vi "Build UDP Payload.vi"(8 "error in (no error)":errorcluster, 11 "DiscoveryService in":refnum<class "NodeDiscovery.lvclass">) -> (0 "error out":errorcluster, 2 "UDP Payload":string, 3 "DiscoveryService out":refnum<class "NodeDiscovery.lvclass">)   [LabVIEW 2020, in "Vecto.lvlib" / "NodeDiscovery.lvclass"]
uses:
  NodeDiscovery.lvclass
  NodeDiscovery.lvclass/NodeDiscovery.ctl
  Vecto.lvlib
  proto/Discovery/Class/Msg.lvclass
  C:/dev/lv20CE/lv-vecto/Vecto/proto/Discovery/Class/Msg.lvclass
  C:/Program Files (x86)/National Instruments/LabVIEW 2020/vi.lib/IlluminatedG/IG Protoc/LV-Proto/Message/Message.lvclass
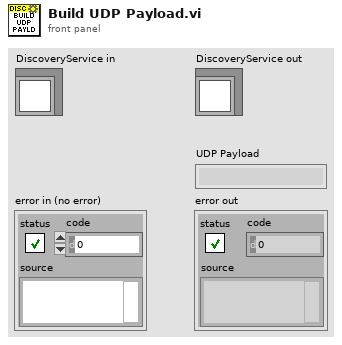
[diagram p1: front panel]
types:
  T1 = typedef "Discovery.lvlib/Data.ctl" = cluster{"node_id":u32, "name":string, "ip":u32, "status":string, "services":T2[], "system":string, "cluster":string}
  T2 = typedef "Service.lvlib/Data.ctl" = cluster{"type":T3, "port":i32}
  T3 = typedef "ServiceType.lvlib/Enumeration.ctl" = enum16{"SERVICETYPE_UNKNOWN", "SERVICETYPE_TCPSERVER", "SERVICETYPE_HTTPSERVER"}
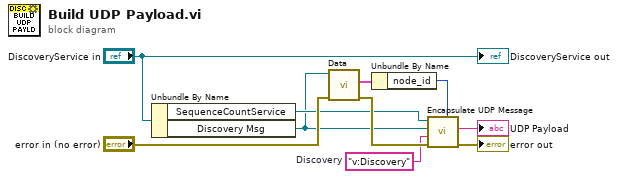
[diagram p0: block diagram]
diagram:
  w1 = "v:Discovery"  # Discovery
  n1 = Unbundle By Name("DiscoveryService in") -> ("SequenceCountService"=w8:refnum<class "SequenceCountService.lvclass">, "Discovery Msg"=w7:refnum<class "Msg.lvclass">)
  n2 = call "Data.vi"("error in (no error)"="error in (no error)", "PB Msg Template in"=w7) -> ("error out"=w10:errorcluster, "Data"=w6:T1)  [unwired: 7 in, 1 out]
  n3 = Unbundle By Name(w6) -> ("node_id"=w5:u32)
  n4 = call "Encapsulate UDP Message.vi"("source_id"=w5, "error in (no error)"=w10, "type"=w1, "Encapsulated Msg"=w7, "SequenceCountService"=w8) -> ("error out"=→"error out":errorcluster, "UDP Payload"=→"UDP Payload":string)  [unwired: 5 in]
  "DiscoveryService out" <- "DiscoveryService in"
